vi "Build.vi"(8 "error in (no error)":errorcluster, 11 "Builder in":refnum<class "Builder.lvclass">) -> (0 "error out":errorcluster, 2 "Built PPL Path":path, 3 "Builder out":refnum<class "Builder.lvclass">)   [LabVIEW 2019, in "Builder.lvclass"]
uses:
  Builder.lvclass
  Builder.lvclass/Builder.ctl
  <vilib>/AppBuilder/AB_API/PPL/NI_AB_API_PPL.lvclass
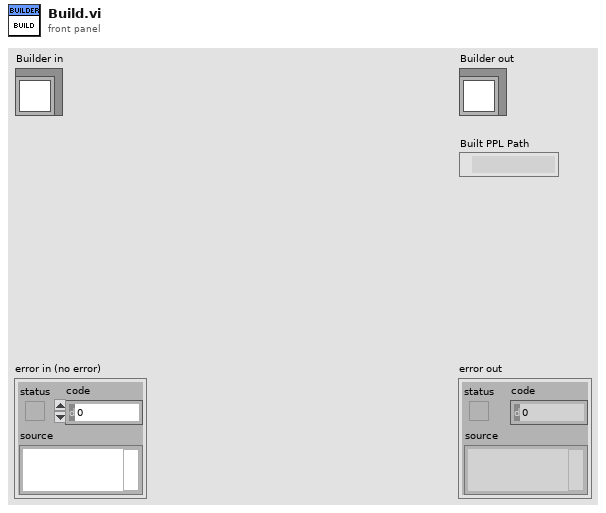
[diagram p1: front panel]
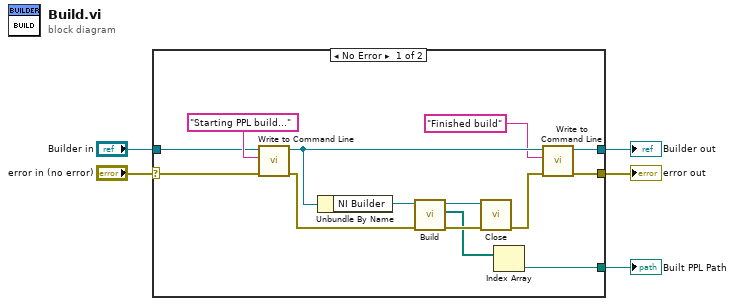
[diagram p0: block diagram]
diagram:
  n1 = case shown="No Error" "error in (no error)" {
    selector: "error in (no error)" -> [w18 w21]
    tunnel: [w9 w21] -> w4
    tunnel: [w8 w20] -> w2
    tunnel: "Builder in" -> [w16 w20]
    tunnel: [w6 _] -> w1
    frame No Error {
      n2 = call "Write to Command Line.vi"("error in (no error)"=w18, "Message"="Starting PPL build...", "Builder in"=w16) -> ("error out"=w14:errorcluster, "Builder out"=w19:refnum<class "Builder.lvclass">)  [unwired: 7 in]
      n3 = Unbundle By Name(w19) -> ("NI Builder"=w15:refnum<class "NI_AB_API_PPL.lvclass">)
      n4 = call-dynamic "Build.vi"("error in (no error)"=w14, "PPL in"=w15) -> ("error out"=w13:errorcluster, "GeneratedFiles"=w12:path[], "PPL out"=w11:refnum<class "NI_AB_API_PPL.lvclass">)  [unwired: 6 in, 1 out]
      n5 = call-dynamic "Close.vi"("error in (no error)"=w13, "DLL in"=w11) -> ("error out"=w10:errorcluster)  [unwired: 9 in]
      n6 = Index Array(array=w12) -> (element=w6:path)  [unwired: 1 in]
      n7 = call "Write to Command Line.vi"("error in (no error)"=w10, "Message"="Finished build", "Builder in"=w19) -> ("error out"=w9:errorcluster, "Builder out"=w8:refnum<class "Builder.lvclass">)  [unwired: 7 in]
    }
    frame Error {
    }
  }
  "error out" <- w4
  "Builder out" <- w2
  "Built PPL Path" <- w1
